vi "Read.vi"(7 "Enable Sound":bool, 8 "error in (no error)":errorcluster, 9 "Audio Channels":cluster{"Left":i32, "Right":i32}, 11 "IntanElectrophysiology in":refnum<class "IntanElectrophysiology.lvclass">) -> (0 "error out":errorcluster, 2 "Samples":u32, 3 "IntanElectrophysiology out":refnum<class "IntanElectrophysiology.lvclass">)   [LabVIEW 2014, in "IntanElectrophysiology.lvclass"]
uses:
  IntanElectrophysiology.lvclass
  IntanElectrophysiology.lvclass/IntanElectrophysiology.ctl
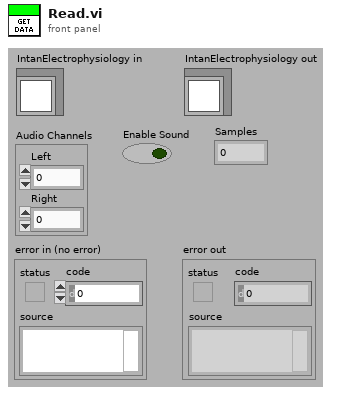
[diagram p1: front panel]
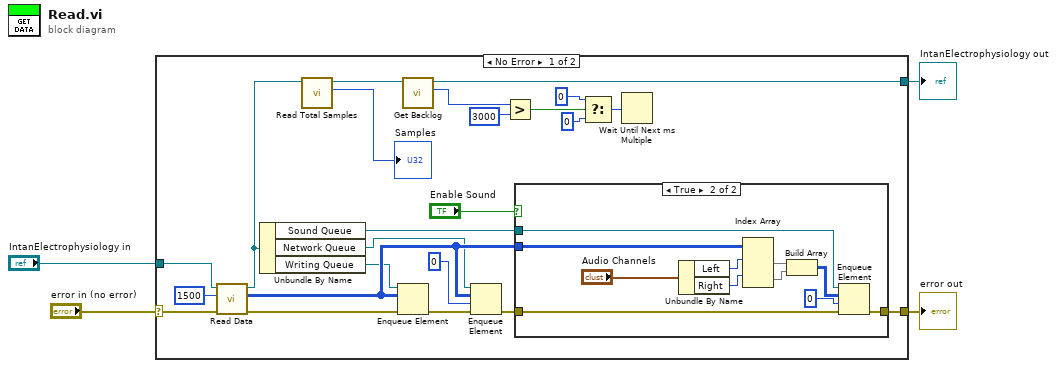
[diagram p0: block diagram]
diagram:
  n1 = case shown="No Error" "error in (no error)" {
    selector: "error in (no error)" -> [w25 w41]
    tunnel: [w27 w41] -> w1
    tunnel: [w9 w40] -> w3
    tunnel: "IntanElectrophysiology in" -> [w26 w40]
    frame No Error {
      n2 = call-dynamic "Read Data.vi"("error in (no error)"=w25, "Read Size"=1500, "IntanElectrophysiology in"=w26) -> ("error out"=w24:errorcluster, "data"=w23:i32[][], "IntanElectrophysiology out"=w5:refnum<class "IntanElectrophysiology.lvclass">)  [unwired: 6 in]
      n3 = Unbundle By Name(w5) -> ("Sound Queue"=w17:refnum<queue>, "Network Queue"=w21:refnum<queue>, "Writing Queue"=w20:refnum<queue>)
      n4 = call-dynamic "Read Total Samples.vi"("AcquireTraces in"=w5) -> ("Total Samples"=→"Samples":u64, "AcquireTraces out"=w10:refnum<class "IntanElectrophysiology.lvclass">)  [unwired: 8 in, 1 out]
      n5 = Enqueue Element(queue=w20, element=w23, error in (no error)=w24) -> (error out=w19:errorcluster)  [unwired: 1 in, 2 out]
      n6 = call-dynamic "Get Backlog.vi"("IntanElectrophysiology in"=w10) -> ("Backlog"=w8:u32, "IntanElectrophysiology out"=w9:refnum<class "IntanElectrophysiology.lvclass">)  [unwired: 8 in, 1 out]
      n7 = Enqueue Element(queue=w21, element=w23, timeout in ms (-1)=0, error in (no error)=w19) -> (error out=w18:errorcluster)  [unwired: 2 out]
      n8 = Greater?(x=w8, y=u32 3000) -> (0:w14:bool)
      n9 = case shown="True" "Enable Sound" {
        tunnel: w17 -> [_ w38]
        tunnel: w18 -> [w28 w37]
        tunnel: [w28 w35] -> w27
        tunnel: w23 -> [_ w34]
        frame False {
        }
        frame True {
          n10 = Unbundle By Name("Audio Channels") -> ("Left"=w39:i32, "Right"=w31:i32)
          n11 = Index Array(array=w34, index (row) #1=w39, index (row) #2=w31) -> (element #1=w32:i32[], element #2=w30:i32[])  [unwired: 2 in]
          n12 = Build Array(w32, w30) -> (w33:i32[][])
          n13 = Enqueue Element(queue=w38, element=w33, timeout in ms (-1)=0, error in (no error)=w37) -> (error out=w35:errorcluster)  [unwired: 2 out]
        }
      }
      n14 = Select(t=0, s=w14, f=u32 0 ("millisecond multiple")) -> (s? t:f=w11:u32)
      n15 = Wait Until Next ms Multiple(millisecond multiple=w11) -> ()  [unwired: 1 out]
    }
    frame Error {
    }
  }
  "error out" <- w1
  "IntanElectrophysiology out" <- w3
